vi "Add Current Sense card.vi"(8 "error in (no error)":errorcluster, 11 "Node Ptr":u64 format="%.0x") -> (0 "error out":errorcluster)   [LabVIEW 2014, in "SLSC configuration System Explorer.lvlib"]
uses:
  SLSC configuration System Explorer.lvlib
  Shared/Constants.vi
  Shared/SLSC configuration Shared.lvlib
panel:
  in  "Tag":string
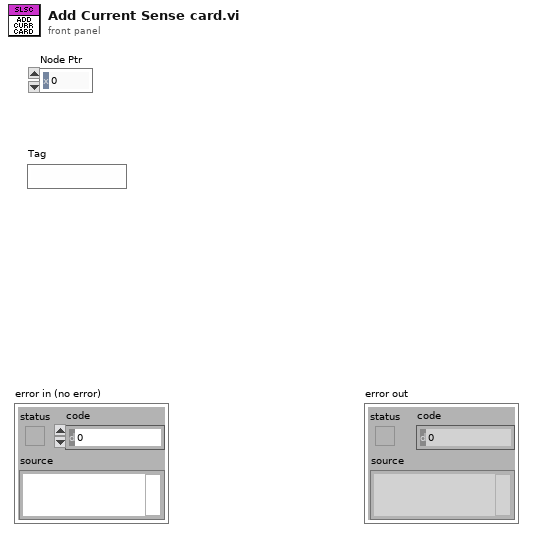
[diagram p1: front panel]
types:
  T1 = typedef "SLSC configuration Shared.lvlib/Card Position.ctl" = cluster{"Rack #":u8, "Slot #":T2}
  T2 = typedef "SLSC configuration Shared.lvlib/Slot #.ctl" = u8
  T3 = typedef "Custom Device API.lvlib/Custom Device Item Ref.ctl" = u64
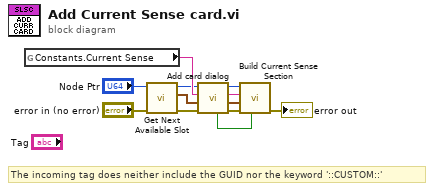
[diagram p0: block diagram]
diagram:
  # "The incoming tag does neither include the GUID nor the keyword '::CUSTOM::'"
  n1 = global read "Constants.vi" "Constants.Current Sense"() -> (w12:string)
  n2 = call "Get Next Available Slot.vi"("error in (no error)"="error in (no error)", "Device Ref in"="Node Ptr") -> ("error out"=w10:errorcluster, "Next Open Slot"=w7:T1, "Device Ref out"=w8:T3)  [unwired: 7 in]
  n3 = call "Add card dialog.vi"("error in (no error)"=w10, "Card Position"=w7, "Card Type in"=w12, "Node Ptr"=w8) -> ("error out"=w3:errorcluster, "Card Position out"=w4:T1, "Name out"=w5:string, "Node Ptr out"=w6:u64, "Cancelled?"=w2:bool)  [unwired: 3 in]
  n4 = call "Build Current Sense Section.vi"("Cancelled?"=w2, "error in (no error)"=w3, "Card Position in"=w4, "Name in"=w5, "Node Ptr in"=w6) -> ("error out"=→"error out":errorcluster)  [unwired: 6 in]
